vi "Measurement.vi"(8 "error in (no error)":errorcluster, 9 "Grandeza":string, 10 "Multiplicador":dbl, 11 "34410A in":refnum<class "34410A.lvclass">) -> (0 "error out":errorcluster, 2 "Measurement":dbl, 3 "34410A out":refnum<class "34410A.lvclass">)   [LabVIEW 2015, in "34410A.lvclass"]
doc: "VI used to measure Value using the multimeter"
uses:
  34410A.lvclass
  <instrlib>/Agilent 34401/Public/Data/Read (Single Point).vi
  <instrlib>/Agilent 34401/Agilent 34401.lvlib
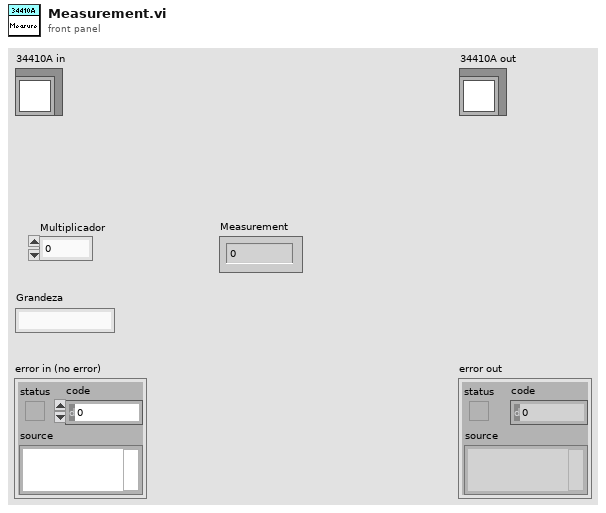
[diagram p1: front panel]
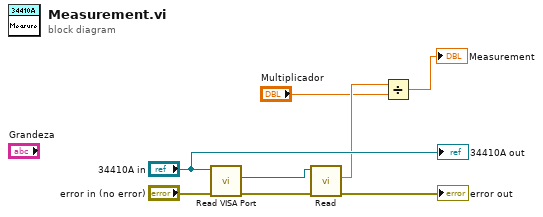
[diagram p0: block diagram]
diagram:
  n1 = call-dynamic "Read VISA Port.vi"("error in (no error)"="error in (no error)", "Device in"="34410A in") -> ("error out"=w7:errorcluster, "VISA Port"=w6:refnum<visa-resource-name>)  [unwired: 7 in, 1 out]
  n2 = call-poly <instrlib>:"Read.vi"("error in (no error)"=w7, "VISA resource name"=w6) -> ("error out"=→"error out":errorcluster, "Measurement"=w3:dbl)  [unwired: 7 in, 1 out]
  n3 = Divide(x=w3, y="Multiplicador") -> (x/y=→"Measurement":dbl)
  "34410A out" <- "34410A in"
